vi "Queue Command.vi"(8 "error in (no error)":errorcluster, 9 "Check Throttle":bool, 10 "Command in":refnum<class "Command Actor.lvclass">, 11 "Command Processor Actor in":refnum<class "Command Processor Actor.lvclass">) -> (0 "error out":errorcluster, 1 "Command Throttled":bool, 2 "Command out":refnum<class "Command Actor.lvclass">, 3 "Command Processor Actor out":refnum<class "Command Processor Actor.lvclass">)   [LabVIEW 2014, in "Robot Actor Framework.lvlib" / "Command Processor Actor.lvlib" / "Command Processor Actor.lvclass"]
uses:
  Command Processor Actor.lvclass
  Command Actor/Command Actor Class/Command Actor.lvclass
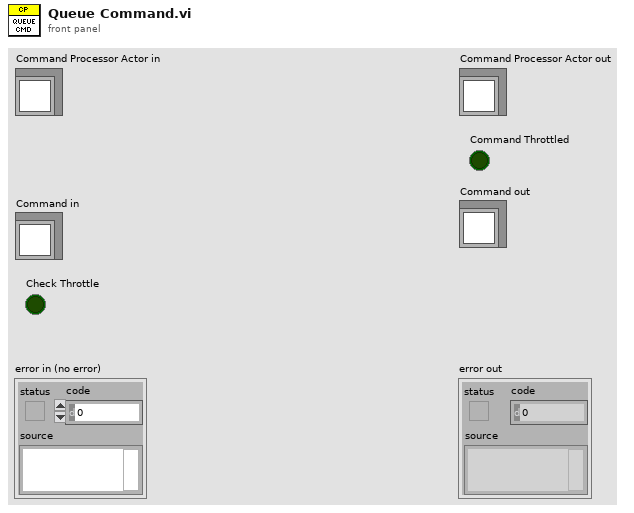
[diagram p1: front panel]
types:
  T1 = enum16{"Critical", "Error", "Warning", "Informational", "Debug"}
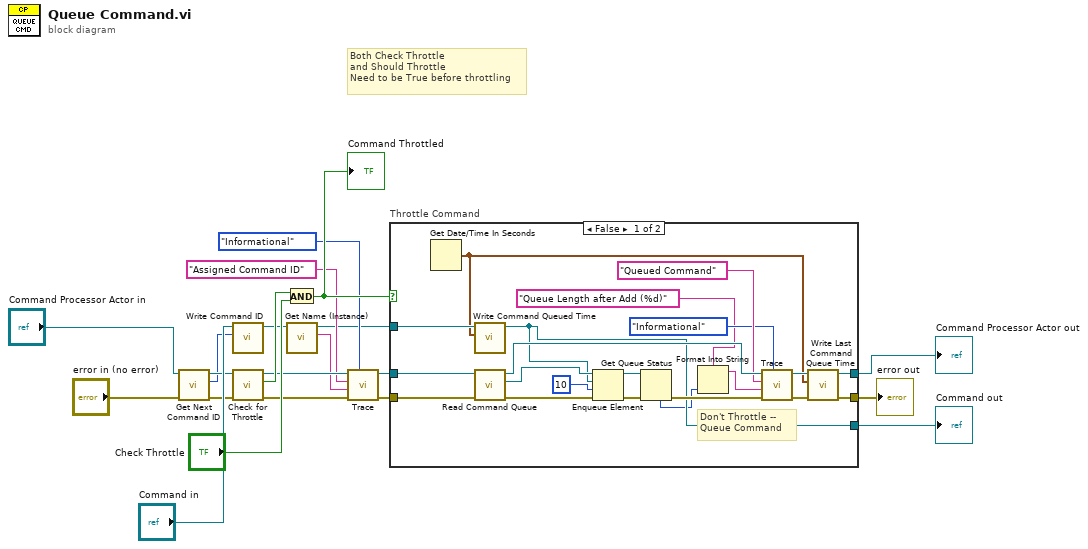
[diagram p0: block diagram]
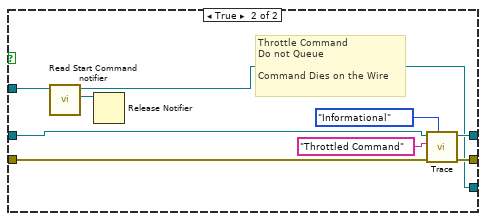
[diagram p2: hidden frame]
diagram:
  # "Both Check Throttle \nand Should Throttle\nNeed to be True before throttling"
  n1 = call-dynamic "Get Next Command ID.vi"("error in (no error)"="error in (no error)", "Command Processor Actor in"="Command Processor Actor in") -> ("error out"=w14:errorcluster, "Next Command ID"=w10:u32, "Command Processor Actor out"=w15:refnum<class "Command Processor Actor.lvclass">)  [unwired: 7 in]
  n2 = call-dynamic "Write Command ID.vi"("Command ID"=w10, "Command in"="Command in") -> ("Command out"=w3:refnum<class "Command Actor.lvclass">)  [unwired: 8 in, 1 out]
  n3 = call-dynamic "Check for Throttle.vi"("error in (no error)"=w14, "Command Processor Actor in"=w15) -> ("error out"=w7:errorcluster, "Should Throttle"=w13:bool, "Command Processor Actor out"=w9:refnum<class "Command Processor Actor.lvclass">)  [unwired: 7 in]
  n4 = And(x=w13, y="Check Throttle") -> (x .and. y?=w11:bool)
  "Command Throttled" <- w11
  n5 = call-dynamic "Get Name (Instance).vi"("Command Actor in"=w3) -> ("Name (Instance)"=w2:string, "Command Actor out"=w1:refnum<class "Command Actor.lvclass">)  [unwired: 8 in, 1 out]
  n6 = call-dynamic "Trace.vi"("Trace Level"=T1."Informational", "error in (no error)"=w7, "Command Processor Message"=w2, "Command Processor Action"="Assigned Command ID", "Command Processor Actor in"=w9) -> ("error out"=w6:errorcluster, "Command Processor Actor out"=w8:refnum<class "Command Processor Actor.lvclass">)  [unwired: 5 in]
  n7 = case "Throttle Command" shown="False" w11 {
    tunnel: w1 -> [w27 w45]
    tunnel: w8 -> [w40 w51]
    tunnel: [w37 w50] -> w19
    tunnel: [w36 w46] -> w17
    tunnel: [w26 w44] -> w16
    tunnel: w6 -> [w34 w47]
    frame False {
      # "Don't Throttle -- \nQueue Command"
      n8 = Get Date/Time In Seconds() -> (seconds since 1Jan1904=w25:timestamp)
      n9 = call-dynamic "Write Command Queued Time.vi"("Command Queued Time"=w25, "Command Actor in"=w27) -> ("Command Actor out"=w26:refnum<class "Command Actor.lvclass">)  [unwired: 8 in, 1 out]
      n10 = call-dynamic "Read Command Queue.vi"("error in (no error)"=w34, "Command Processor Actor in"=w40) -> ("error out"=w42:errorcluster, "Queued Commands"=w39:refnum<queue>, "Command Processor Actor out"=w33:refnum<class "Command Processor Actor.lvclass">)  [unwired: 7 in]
      n11 = Enqueue Element(queue=w39, element=w26, timeout in ms (-1)=10, error in (no error)=w42) -> (queue out=w38:refnum<queue>, error out=w41:errorcluster)  [unwired: 1 out]
      n12 = Get Queue Status(queue=w38, error in (no error)=w41) -> (error out=w31:errorcluster, # elements in queue=w23:i32)  [unwired: 1 in, 6 out]
      n13 = Format Into String(format string="Queue Length after Add (%d)", w23) -> (resulting string=w22:string)  [unwired: 2 in, 1 out]
      n14 = call-dynamic "Trace.vi"("Trace Level"=T1."Informational", "error in (no error)"=w31, "Command Processor Message"=w22, "Command Processor Action"="Queued Command", "Command Processor Actor in"=w33) -> ("error out"=w30:errorcluster, "Command Processor Actor out"=w32:refnum<class "Command Processor Actor.lvclass">)  [unwired: 5 in]
      n15 = call-dynamic "Write Last Command Queue Time.vi"("error in (no error)"=w30, "Last Command Queue Time"=w25, "Command Processor Actor in"=w32) -> ("error out"=w36:errorcluster, "Command Processor Actor out"=w37:refnum<class "Command Processor Actor.lvclass">)  [unwired: 7 in]
    }
    frame True {
      # "Throttle Command\nDo not Queue\n\nCommand Dies on the Wire"
      n16 = call-dynamic "Read Start Command notifier.vi"("Command Actor in"=w45) -> ("Command Stop notifier"=w43:refnum<notifier>, "Command Actor out"=w44:refnum<class "Command Actor.lvclass">)  [unwired: 8 in, 1 out]
      n17 = Release Notifier(notifier=w43) -> ()  [unwired: 2 in, 3 out]
      n18 = call-dynamic "Trace.vi"("Trace Level"=T1."Informational", "error in (no error)"=w47, "Command Processor Action"="Throttled Command", "Command Processor Actor in"=w51) -> ("error out"=w46:errorcluster, "Command Processor Actor out"=w50:refnum<class "Command Processor Actor.lvclass">)  [unwired: 6 in]
    }
  }
  "error out" <- w17
  "Command Processor Actor out" <- w19
  "Command out" <- w16
